vi "sub_result-update.vi"   [LabVIEW 2019]
uses:
  _ctrl/rw.ctl
  SubVIs/common/_ctrl/system-status.ctl
  SubVIs/common/Glob_Ref.vi
types:
  T1 = typedef "rw.ctl" = enum16{"read", "write"}
  T2 = typedef "DL950_wfms.ctl" = cluster{"wfms":waveform(dbl)[], "Waveform_2":cluster{"t0":dbl, "dt":dbl, "Y":dbl[][]}, "items":dbl[][], "da950_array":dbl[]}
  T3 = typedef "Testing-info.ctl" = cluster{"전체채널수":u8, "현재채널번호":u8, "Irms":dbl, "입력전압":dbl, "입력전류":dbl, "출력전압":dbl, "출력전류":dbl, "온도":dbl, "제어단 단선":bool, "제어단 단락":bool, "제어단 특성변화":bool, "출력단 단선":bool, "출력단 단락":bool, "출력단 특성변화":bool, "출력단 전압":bool, "카운트 일치":bool, "Irms 판정":bool, "온도":bool, "테스트 회수":u32, "TestType":T4, "현재회수":u32, "Ch selection":cluster{"1ch":bool, "2ch":bool, "3ch":bool, "4ch":bool, "5ch":bool, "6ch":bool}, "반복":u32, "Path":path, "파일생성주기":u32, "start time":dbl, "stop time":dbl, "현재반복회수":u32, "NG":cluster{"입출력 카운트":bool, "출력전류RMS":bool}}
  T4 = typedef "sequence_single.ctl" = enum16{"Register", "RC", "B1", "B2", "B3", "Oper_LV", "Oper_HV", "ContR_LV"}
  T5 = typedef "system-status.ctl" = enum16{"Initial", "Update", "Clear", "Read"}
  T6 = typedef "measure_reg.ctl" = cluster{"입력카운트":dbl, "출력카운트":dbl, "부하전압 RMS":dbl, "입력전류 RMS":dbl, "출력전류 RMS":dbl, "온도":dbl, "부하전압(고장)":dbl}
  T7 = typedef "measure_rc.ctl" = cluster{"입력카운트":dbl, "출력카운트":dbl, "Rising Time 63%":dbl, "Rising Time 98%":dbl, "Failing Time 37%":dbl, "입력전류 RMS":dbl, "출력전류 RMS":dbl, "출력전압 + 평균 63%":dbl, "출력전압 - 평균 63%":dbl, "출력전류 평균 63%":dbl, "접촉저항":dbl, "온도":dbl, "충전전압 63초":dbl, "충전전압 98초":dbl, "충전전류 37초":dbl, "방전전압":dbl, "전압강하":dbl, "부하전압(고장)":dbl}
  T8 = typedef "data_contR.ctl" = cluster{"입력카운트":dbl, "출력카운트":dbl, "입력전류 RMS":dbl, "출력전류 RMS":dbl, "출력전압(+)_Avg":dbl, "출력전압(-)_Avg":dbl, "출력전류_Avg":dbl, "접촉저항":dbl, "온도":dbl, "부하전압":dbl}
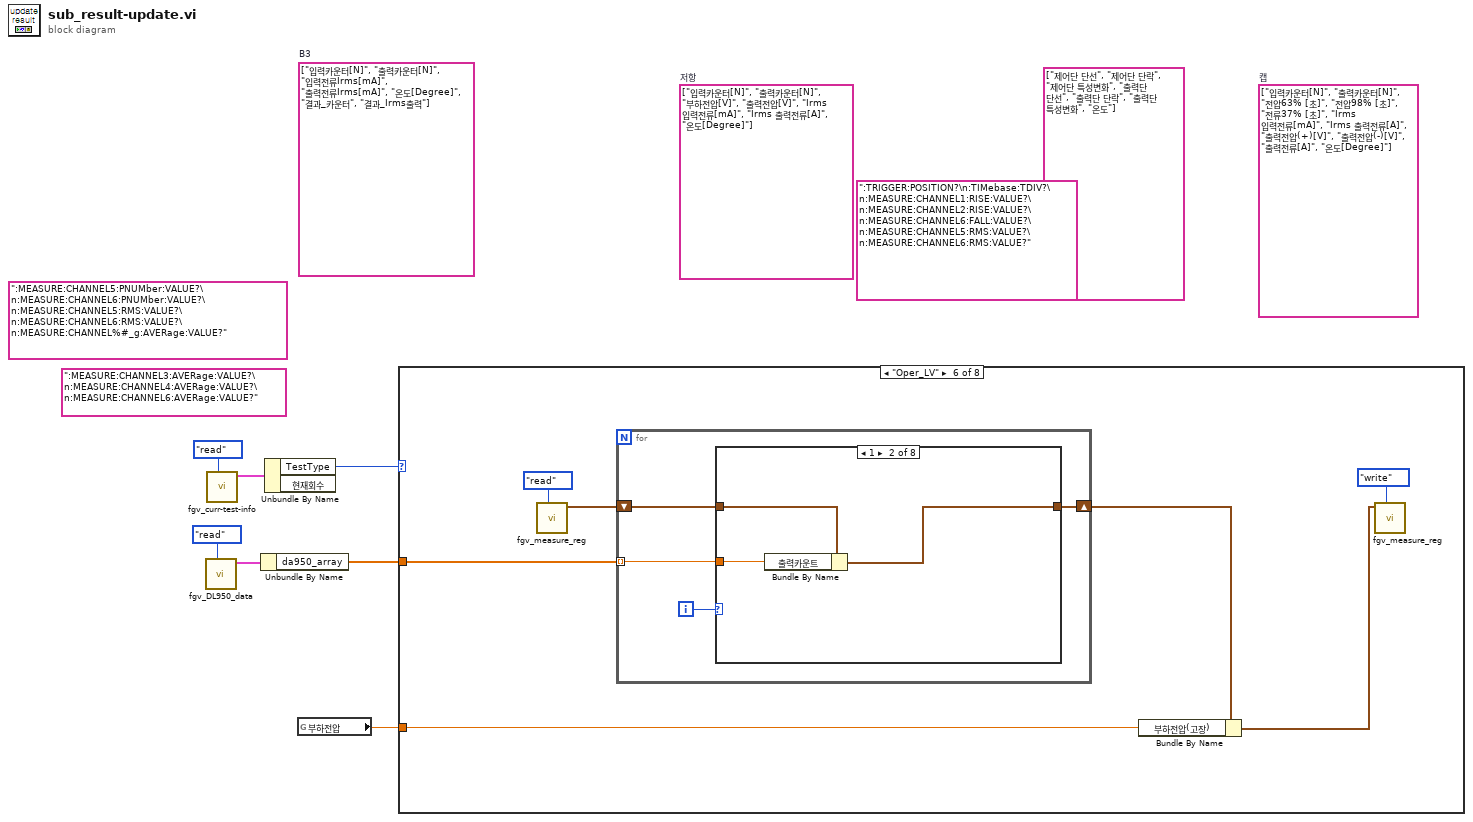
[diagram p0: block diagram]
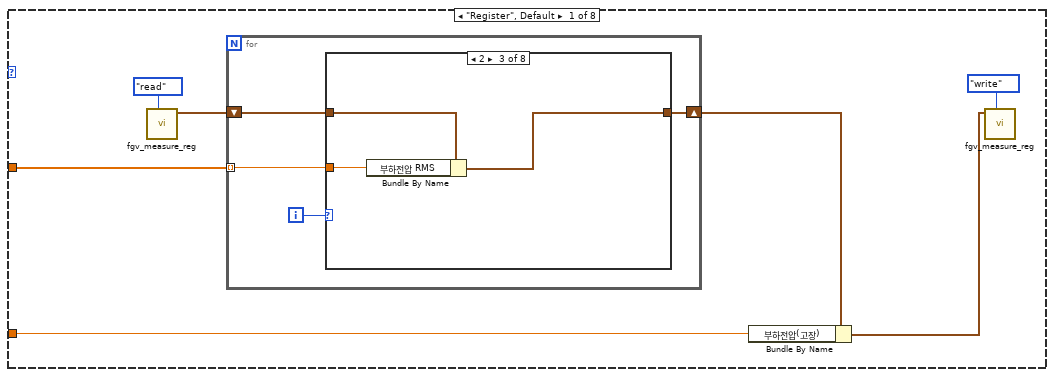
[diagram p2: hidden frame]
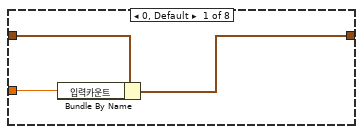
[diagram p3: hidden frame]
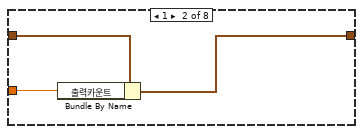
[diagram p4: hidden frame]
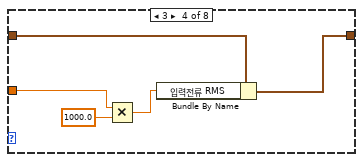
[diagram p5: hidden frame]
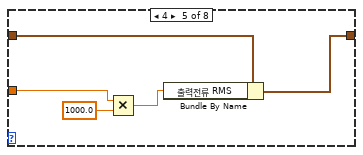
[diagram p6: hidden frame]
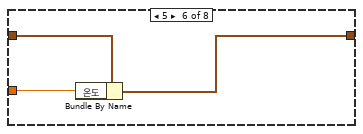
[diagram p7: hidden frame]
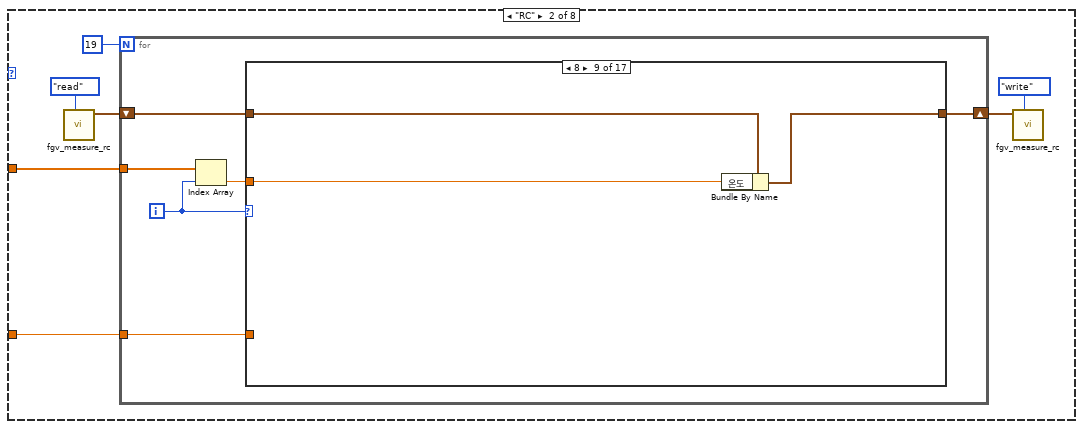
[diagram p10: hidden frame]
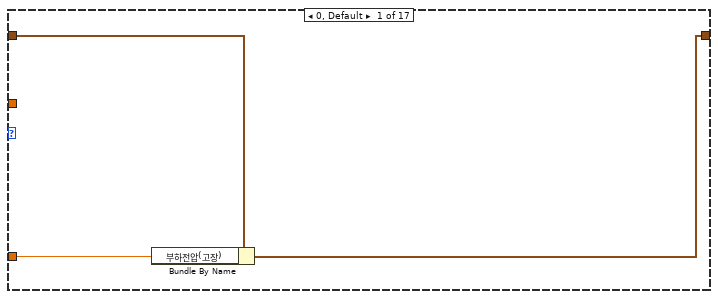
[diagram p11: hidden frame]
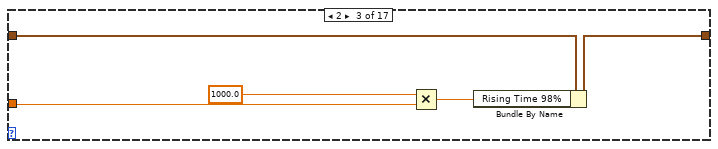
[diagram p13: hidden frame]
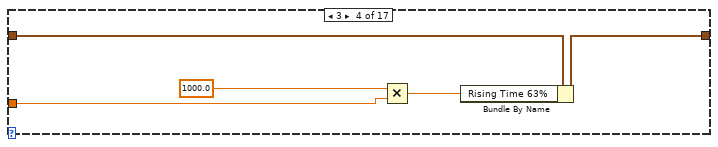
[diagram p14: hidden frame]
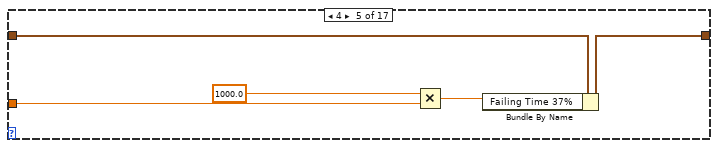
[diagram p15: hidden frame]
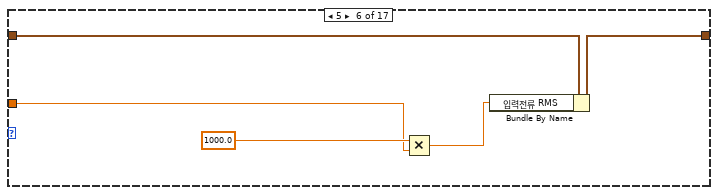
[diagram p16: hidden frame]
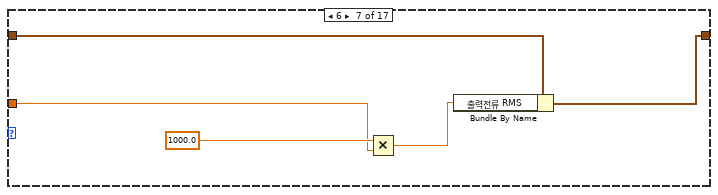
[diagram p17: hidden frame]
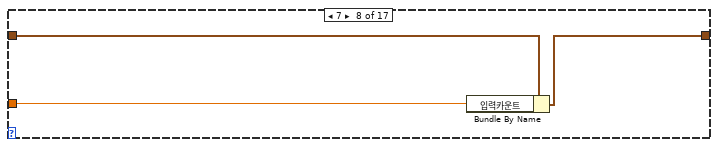
[diagram p18: hidden frame]
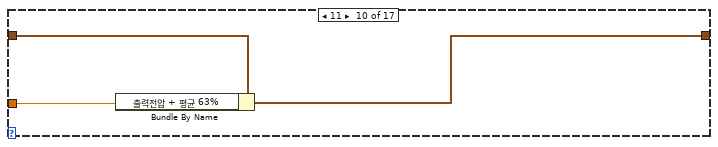
[diagram p19: hidden frame]
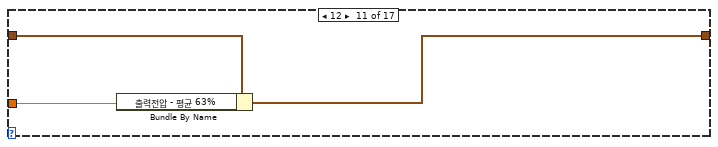
[diagram p20: hidden frame]
diagram:
  (unwired) ":MEASURE:CHANNEL3:AVERage:VALUE?\n:MEASURE:CHANNEL4:AVERage:VALUE?\n:MEASURE:CHANNEL6:AVERage:VALUE?" ("String")
  (unwired) ":MEASURE:CHANNEL5:PNUMber:VALUE?\n:MEASURE:CHANNEL6:PNUMber:VALUE?\n:MEASURE:CHANNEL5:RMS:VALUE?\n:MEASURE:CHANNEL6:RMS:VALUE?\n:MEASURE:CHANNEL%#_g:AVERage:VALUE?" ("String")
  (unwired) string[] ["입력카운터[N]", "출력카운터[N]", "입력전류Irms[mA]", "출력전류Irms[mA]", "온도[Degree]", "결과_카운터", "결과_Irms출력"]  # B3
  (unwired) ":TRIGGER:POSITION?\n:TIMebase:TDIV?\n:MEASURE:CHANNEL1:RISE:VALUE?\n:MEASURE:CHANNEL2:RISE:VALUE?\n:MEASURE:CHANNEL6:FALL:VALUE?\n:MEASURE:CHANNEL5:RMS:VALUE?\n:MEASURE:CHANNEL6:RMS:VALUE?" ("String")
  (unwired) string[] ["제어단 단선", "제어단 단락", "제어단 특성변화", "출력단 단선", "출력단 단락", "출력단 특성변화", "온도"] ("Column Header Strings[]")
  (unwired) string[] ["입력카운터[N]", "출력카운터[N]", "전압63% [초]", "전압98% [초]", "전류37% [초]", "Irms 입력전류[mA]", "Irms 출력전류[A]", "출력전압(+)[V]", "출력전압(-)[V]", "출력전류[A]", "온도[Degree]"]  # 캡
  (unwired) string[] ["입력카운터[N]", "출력카운터[N]", "부하전압[V]", "출력전압[V]", "Irms 입력전류[mA]", "Irms 출력전류[A]", "온도[Degree]"]  # 저항
  n1 = call "fgv_DL950_data.vi"("cmd"=rw."read") -> ("DL950 wfm 2"=w3:T2)  [unwired: 9 in, 1 out]
  n2 = call "fgv_curr-test-info.vi"("cmd"=rw."read") -> ("현재테스트 정보 2"=w5:T3)  [unwired: 10 in]
  n3 = Unbundle By Name(w3) -> ("da950_array"=w4:dbl[])
  n4 = Unbundle By Name(w5) -> ("TestType"=w7:T4)  [unwired: 1 out]
  n5 = global read "Glob_Ref.vi" "부하전압"() -> (w1:dbl)
  n6 = case shown="\"Oper_LV\"" w7 {
    tunnel: w4 -> [w14 w47 w132 w218 w253 w288 w331 w376]
    tunnel: w1 -> [w8 w43 w128 w212 w248 w282 w330 w372]
    frame "Register", Default {
      n7 = call "fgv_measure_reg.vi"("cmd"=rw."read") -> ("measure_reg 2"=w12:T6)  [unwired: 10 in]
      n8 = for {
        tunnel: w14 -> [w15] mode=indexing
        shift-right: [w16] -> w10
        shift-left: w12 -> [w17]
        i -> [w18]
        n9 = case shown="2" w18 {
          tunnel: w17 -> [w21 w24 w27 w32 w37 w40 w41 w42]
          tunnel: [w20 w23 w26 w31 w36 w39 w41 w42] -> w16
          tunnel: w15 -> [w19 w22 w25 w30 w34 w38 _ _]
          frame 0, Default {
            n10 = Bundle By Name(cluster=w21, "입력카운트"=w19) -> (w20:T6)
          }
          frame 1 {
            n11 = Bundle By Name(cluster=w24, "출력카운트"=w22) -> (w23:T6)
          }
          frame 2 {
            n12 = Bundle By Name(cluster=w27, "부하전압 RMS"=w25) -> (w26:T6)
          }
          frame 3 {
            n13 = Multiply(x=w30, y=1000.0) -> (x*y=w29:dbl)
            n14 = Bundle By Name(cluster=w32, "입력전류 RMS"=w29) -> (w31:T6)
          }
          frame 4 {
            n15 = Multiply(x=w34, y=1000.0) -> (x*y=w33:dbl)
            n16 = Bundle By Name(cluster=w37, "출력전류 RMS"=w33) -> (w36:T6)
          }
          frame 5 {
            n17 = Bundle By Name(cluster=w40, "온도"=w38) -> (w39:T6)
          }
          frame 6 {
          }
          frame 7 {
          }
        }
      }
      n18 = Bundle By Name(cluster=w10, "부하전압(고장)"=w8) -> (w9:T6)
      n19 = call "fgv_measure_reg.vi"("cmd"=rw."write", "measure_reg"=w9) -> ()  [unwired: 9 in, 1 out]
    }
    frame "RC" {
      n20 = call "fgv_measure_rc.vi"("cmd"=rw."read") -> ("measure_rc 2"=w46:T7)  [unwired: 10 in]
      n21 = for {
        N: 19 -> [_]
        tunnel: w47 -> [w55]
        shift-right: [w50] -> w45
        shift-left: w46 -> [w54]
        tunnel: w43 -> [w51]
        i -> [w52]
        n22 = Index Array(array=w55, index=w52) -> (element=w53:dbl)
        n23 = case shown="8" w52 {
          tunnel: w54 -> [w58 w59 w64 w69 w74 w79 w81 w87 w90 w92 w95 w98 w104 w105 w106 w124 w127]
          tunnel: [w57 w59 w63 w68 w73 w78 w80 w86 w89 w91 w94 w97 w103 w105 w106 w125 w127] -> w50
          tunnel: w53 -> [_ _ w62 w66 w71 w76 w82 w85 w88 w93 w96 w99 _ _ _ _ _]
          tunnel: w51 -> [w56 _ _ _ _ _ _ _ _ _ _ _ _ _ _ _ _]
          frame 0, Default {
            n24 = Bundle By Name(cluster=w58, "부하전압(고장)"=w56) -> (w57:T7)
          }
          frame 1 {
          }
          frame 2 {
            n25 = Multiply(x=1000.0, y=w62) -> (x*y=w61:dbl)
            n26 = Bundle By Name(cluster=w64, "Rising Time 98%"=w61) -> (w63:T7)
          }
          frame 3 {
            n27 = Multiply(x=1000.0, y=w66) -> (x*y=w65:dbl)
            n28 = Bundle By Name(cluster=w69, "Rising Time 63%"=w65) -> (w68:T7)
          }
          frame 4 {
            n29 = Multiply(x=1000.0, y=w71) -> (x*y=w70:dbl)
            n30 = Bundle By Name(cluster=w74, "Failing Time 37%"=w70) -> (w73:T7)
          }
          frame 5 {
            n31 = Multiply(x=1000.0, y=w76) -> (x*y=w75:dbl)
            n32 = Bundle By Name(cluster=w79, "입력전류 RMS"=w75) -> (w78:T7)
          }
          frame 6 {
            n33 = Multiply(x=1000.0, y=w82) -> (x*y=w83:dbl)
            n34 = Bundle By Name(cluster=w81, "출력전류 RMS"=w83) -> (w80:T7)
          }
          frame 7 {
            n35 = Bundle By Name(cluster=w87, "입력카운트"=w85) -> (w86:T7)
          }
          frame 8 {
            n36 = Bundle By Name(cluster=w90, "온도"=w88) -> (w89:T7)
          }
          frame 11 {
            n37 = Bundle By Name(cluster=w92, "출력전압 + 평균 63%"=w93) -> (w91:T7)
          }
          frame 12 {
            n38 = Bundle By Name(cluster=w95, "출력전압 - 평균 63%"=w96) -> (w94:T7)
          }
          frame 13 {
            n39 = Bundle By Name(cluster=w98, "출력전류 평균 63%"=w99) -> (w97:T7)
          }
          frame 14 {
            n40 = call "fgv_AI.vi"("Mode"=system-status."Read") -> ("mean-vals"=w101:dbl[])  [unwired: 8 in, 2 out]
            n41 = Index Array(array=w101) -> (element=w100:dbl)  [unwired: 1 in]
            n42 = Bundle By Name(cluster=w104, "방전전압"=w100) -> (w103:T7)
          }
          frame 15 {
          }
          frame 16 {
          }
          frame 18 {
            n43 = Unbundle By Name(w124) -> ("출력전압 + 평균 63%"=w112:dbl, "출력전압 - 평균 63%"=w109:dbl, "출력전류 평균 63%"=w116:dbl)
            n44 = Number To Fractional String(number=w109) -> (F-format string=w111:string)  [unwired: 3 in]
            n45 = Number To Fractional String(number=w112) -> (F-format string=w113:string)  [unwired: 3 in]
            n46 = call "sub_log_basic.vi"("desc"=w113, "Title"="output volt+ 63%") -> ("error out"=w108:errorcluster)  [unwired: 9 in]
            n47 = call "sub_log_basic.vi"("error in"=w108, "desc"=w111, "Title"="output volt- 63%") -> ("error out"=w107:errorcluster)  [unwired: 8 in]
            n48 = Subtract(x=w112, y=w109) -> (x-y=w126:dbl)
            n49 = Divide(x=w126, y=w116) -> (x/y=w122:dbl)
            n50 = Number To Fractional String(number=w116) -> (F-format string=w118:string)  [unwired: 3 in]
            n51 = Multiply(x=1000.0, y=w122) -> (x*y=w120:dbl)
            n52 = call "sub_log_basic.vi"("error in"=w107, "desc"=w118, "Title"="output current 63%") -> ("error out"=w115:errorcluster)  [unwired: 8 in]
            n53 = Bundle By Name(cluster=w124, "접촉저항"=w120) -> (w125:T7)
            n54 = Number To Fractional String(number=w120) -> (F-format string=w119:string)  [unwired: 3 in]
            n55 = call "sub_log_basic.vi"("error in"=w115, "desc"=w119, "Title"="contact register") -> ()  [unwired: 8 in, 1 out]
          }
          frame 19 {
          }
        }
      }
      n56 = call "fgv_measure_rc.vi"("cmd"=rw."write", "measure_rc"=w45) -> ()  [unwired: 9 in, 1 out]
    }
    frame "B1" {
      n57 = call "fgv_measure_rc.vi"("cmd"=rw."read") -> ("measure_rc 2"=w131:T7)  [unwired: 10 in]
      n58 = for {
        N: 19 -> [_]
        tunnel: w132 -> [w138]
        shift-right: [w139] -> w130
        shift-left: w131 -> [w140]
        tunnel: w128 -> [w135]
        i -> [w137]
        n59 = Index Array(array=w138, index=w137) -> (element=w136:dbl)
        n60 = case shown="0, Default" w137 {
          tunnel: w140 -> [w143 w144 w149 w154 w159 w164 w166 w172 w174 w177 w180 w186 w188 w190 w208 w211]
          tunnel: [w141 w144 w148 w153 w158 w163 w165 w171 w173 w176 w179 w185 w187 w190 w209 w211] -> w139
          tunnel: w136 -> [_ _ w147 w151 w156 w161 w167 w170 w175 w178 w181 _ w189 _ _ _]
          tunnel: w135 -> [w142 _ _ _ _ _ _ _ _ _ _ _ _ _ _ _]
          frame 0, Default {
            n61 = Bundle By Name(cluster=w143, "부하전압(고장)"=w142) -> (w141:T7)
          }
          frame 1 {
          }
          frame 2 {
            n62 = Multiply(x=1000.0, y=w147) -> (x*y=w146:dbl)
            n63 = Bundle By Name(cluster=w149, "Rising Time 98%"=w146) -> (w148:T7)
          }
          frame 3 {
            n64 = Multiply(x=1000.0, y=w151) -> (x*y=w150:dbl)
            n65 = Bundle By Name(cluster=w154, "Rising Time 63%"=w150) -> (w153:T7)
          }
          frame 4 {
            n66 = Multiply(x=1000.0, y=w156) -> (x*y=w155:dbl)
            n67 = Bundle By Name(cluster=w159, "Failing Time 37%"=w155) -> (w158:T7)
          }
          frame 5 {
            n68 = Multiply(x=1000.0, y=w161) -> (x*y=w160:dbl)
            n69 = Bundle By Name(cluster=w164, "입력전류 RMS"=w160) -> (w163:T7)
          }
          frame 6 {
            n70 = Multiply(x=1000.0, y=w167) -> (x*y=w168:dbl)
            n71 = Bundle By Name(cluster=w166, "출력전류 RMS"=w168) -> (w165:T7)
          }
          frame 7 {
            n72 = Bundle By Name(cluster=w172, "입력카운트"=w170) -> (w171:T7)
          }
          frame 10 {
            n73 = Bundle By Name(cluster=w174, "출력전압 + 평균 63%"=w175) -> (w173:T7)
          }
          frame 11 {
            n74 = Bundle By Name(cluster=w177, "출력전압 - 평균 63%"=w178) -> (w176:T7)
          }
          frame 12 {
            n75 = Bundle By Name(cluster=w180, "출력전류 평균 63%"=w181) -> (w179:T7)
          }
          frame 13 {
            n76 = call "fgv_AI.vi"("Mode"=system-status."Read") -> ("mean-vals"=w183:dbl[])  [unwired: 8 in, 2 out]
            n77 = Index Array(array=w183) -> (element=w182:dbl)  [unwired: 1 in]
            n78 = Bundle By Name(cluster=w186, "방전전압"=w182) -> (w185:T7)
          }
          frame 15 {
            n79 = Bundle By Name(cluster=w188, "온도"=w189) -> (w187:T7)
          }
          frame 16 {
          }
          frame 18 {
            n80 = Unbundle By Name(w208) -> ("출력전압 + 평균 63%"=w196:dbl, "출력전압 - 평균 63%"=w193:dbl, "출력전류 평균 63%"=w200:dbl)
            n81 = Number To Fractional String(number=w193) -> (F-format string=w195:string)  [unwired: 3 in]
            n82 = Number To Fractional String(number=w196) -> (F-format string=w197:string)  [unwired: 3 in]
            n83 = call "sub_log_basic.vi"("desc"=w197, "Title"="output volt+ 63%") -> ("error out"=w192:errorcluster)  [unwired: 9 in]
            n84 = call "sub_log_basic.vi"("error in"=w192, "desc"=w195, "Title"="output volt- 63%") -> ("error out"=w191:errorcluster)  [unwired: 8 in]
            n85 = Subtract(x=w196, y=w193) -> (x-y=w210:dbl)
            n86 = Divide(x=w210, y=w200) -> (x/y=w206:dbl)
            n87 = Number To Fractional String(number=w200) -> (F-format string=w202:string)  [unwired: 3 in]
            n88 = Multiply(x=1000.0, y=w206) -> (x*y=w204:dbl)
            n89 = call "sub_log_basic.vi"("error in"=w191, "desc"=w202, "Title"="output current 63%") -> ("error out"=w199:errorcluster)  [unwired: 8 in]
            n90 = Bundle By Name(cluster=w208, "접촉저항"=w204) -> (w209:T7)
            n91 = Number To Fractional String(number=w204) -> (F-format string=w203:string)  [unwired: 3 in]
            n92 = call "sub_log_basic.vi"("error in"=w199, "desc"=w203, "Title"="contact register") -> ()  [unwired: 8 in, 1 out]
          }
          frame 19 {
          }
        }
      }
      n93 = call "fgv_measure_rc.vi"("cmd"=rw."write", "measure_rc"=w130) -> ()  [unwired: 9 in, 1 out]
    }
    frame "B2" {
      n94 = call "fgv_measure_reg.vi"("cmd"=rw."read") -> ("measure_reg 2"=w216:T6)  [unwired: 10 in]
      n95 = for {
        tunnel: w218 -> [w219] mode=indexing
        shift-right: [w220] -> w214
        shift-left: w216 -> [w221]
        i -> [w222]
        n96 = case shown="2" w222 {
          tunnel: w221 -> [w225 w228 w231 w236 w241 w244 w245 w246]
          tunnel: [w224 w227 w230 w235 w240 w243 w245 w246] -> w220
          tunnel: w219 -> [w223 w226 w229 w234 w238 w242 _ _]
          frame 0, Default {
            n97 = Bundle By Name(cluster=w225, "입력카운트"=w223) -> (w224:T6)
          }
          frame 1 {
            n98 = Bundle By Name(cluster=w228, "출력카운트"=w226) -> (w227:T6)
          }
          frame 2 {
            n99 = Bundle By Name(cluster=w231, "부하전압 RMS"=w229) -> (w230:T6)
          }
          frame 3 {
            n100 = Multiply(x=w234, y=1000.0) -> (x*y=w233:dbl)
            n101 = Bundle By Name(cluster=w236, "입력전류 RMS"=w233) -> (w235:T6)
          }
          frame 4 {
            n102 = Multiply(x=w238, y=1000.0) -> (x*y=w237:dbl)
            n103 = Bundle By Name(cluster=w241, "출력전류 RMS"=w237) -> (w240:T6)
          }
          frame 5 {
            n104 = Bundle By Name(cluster=w244, "온도"=w242) -> (w243:T6)
          }
          frame 6 {
          }
          frame 7 {
          }
        }
      }
      n105 = Bundle By Name(cluster=w214, "부하전압(고장)"=w212) -> (w213:T6)
      n106 = call "fgv_measure_reg.vi"("cmd"=rw."write", "measure_reg"=w213) -> ()  [unwired: 9 in, 1 out]
    }
    frame "B3" {
      n107 = call "fgv_measure_reg.vi"("cmd"=rw."read") -> ("measure_reg 2"=w251:T6)  [unwired: 10 in]
      n108 = for {
        tunnel: w253 -> [w254] mode=indexing
        shift-right: [w255] -> w249
        shift-left: w251 -> [w256]
        i -> [w257]
        n109 = case shown="0, Default" w257 {
          tunnel: w256 -> [w260 w263 w266 w271 w276 w279 w280 w281]
          tunnel: [w259 w262 w265 w270 w275 w278 w280 w281] -> w255
          tunnel: w254 -> [w258 w261 w264 w269 w273 w277 _ _]
          frame 0, Default {
            n110 = Bundle By Name(cluster=w260, "입력카운트"=w258) -> (w259:T6)
          }
          frame 1 {
            n111 = Bundle By Name(cluster=w263, "출력카운트"=w261) -> (w262:T6)
          }
          frame 2 {
            n112 = Bundle By Name(cluster=w266, "부하전압 RMS"=w264) -> (w265:T6)
          }
          frame 3 {
            n113 = Multiply(x=w269, y=1000.0) -> (x*y=w268:dbl)
            n114 = Bundle By Name(cluster=w271, "입력전류 RMS"=w268) -> (w270:T6)
          }
          frame 4 {
            n115 = Multiply(x=w273, y=1000.0) -> (x*y=w272:dbl)
            n116 = Bundle By Name(cluster=w276, "출력전류 RMS"=w272) -> (w275:T6)
          }
          frame 5 {
            n117 = Bundle By Name(cluster=w279, "온도"=w277) -> (w278:T6)
          }
          frame 6 {
          }
          frame 7 {
          }
        }
      }
      n118 = Bundle By Name(cluster=w249, "부하전압(고장)"=w248) -> (w247:T6)
      n119 = call "fgv_measure_reg.vi"("cmd"=rw."write", "measure_reg"=w247) -> ()  [unwired: 9 in, 1 out]
    }
    frame "Oper_LV" {
      n120 = call "fgv_measure_reg.vi"("cmd"=rw."read") -> ("measure_reg 2"=w286:T6)  [unwired: 10 in]
      n121 = for {
        tunnel: w288 -> [w289] mode=indexing
        shift-right: [w290] -> w284
        shift-left: w286 -> [w291]
        i -> [w292]
        n122 = case shown="1" w292 {
          tunnel: w291 -> [w295 w298 w301 w306 w311 w314 w315 w316]
          tunnel: [w294 w297 w300 w305 w310 w313 w315 w316] -> w290
          tunnel: w289 -> [w293 w296 w299 w304 w308 w312 _ _]
          frame 0, Default {
            n123 = Bundle By Name(cluster=w295, "입력카운트"=w293) -> (w294:T6)
          }
          frame 1 {
            n124 = Bundle By Name(cluster=w298, "출력카운트"=w296) -> (w297:T6)
          }
          frame 2 {
            n125 = Bundle By Name(cluster=w301, "부하전압 RMS"=w299) -> (w300:T6)
          }
          frame 3 {
            n126 = Multiply(x=w304, y=1000.0) -> (x*y=w303:dbl)
            n127 = Bundle By Name(cluster=w306, "입력전류 RMS"=w303) -> (w305:T6)
          }
          frame 4 {
            n128 = Multiply(x=w308, y=1000.0) -> (x*y=w307:dbl)
            n129 = Bundle By Name(cluster=w311, "출력전류 RMS"=w307) -> (w310:T6)
          }
          frame 5 {
            n130 = Bundle By Name(cluster=w314, "온도"=w312) -> (w313:T6)
          }
          frame 6 {
          }
          frame 7 {
          }
        }
      }
      n131 = Bundle By Name(cluster=w284, "부하전압(고장)"=w282) -> (w283:T6)
      n132 = call "fgv_measure_reg.vi"("cmd"=rw."write", "measure_reg"=w283) -> ()  [unwired: 9 in, 1 out]
    }
    frame "ContR_LV" {
      w318 = 1000.0 ("y")
      n133 = call "fgv_measure_ContR.vi"("cmd"=rw."read") -> ("measure_ContR Out"=w328:T8)  [unwired: 9 in, 1 out]
      n134 = for {
        tunnel: w331 -> [w332] mode=indexing
        shift-right: [w333] -> w325
        shift-left: w328 -> [w334]
        i -> [w335]
        n135 = case shown="11" w335 {
          tunnel: w334 -> [w338 w341 w346 w351 w354 w355 w356 w361 w366 w369 w370 w371]
          tunnel: [w337 w340 w345 w350 w353 w355 w356 w360 w365 w368 w370 w371] -> w333
          tunnel: w332 -> [w336 w339 w343 w349 w352 _ _ w358 w363 w367 _ _]
          frame 0, Default {
            n136 = Bundle By Name(cluster=w338, "입력카운트"=w336) -> (w337:T8)
          }
          frame 1 {
            n137 = Bundle By Name(cluster=w341, "출력카운트"=w339) -> (w340:T8)
          }
          frame 2 {
            n138 = Multiply(x=w343, y=1000.0) -> (x*y=w342:dbl)
            n139 = Bundle By Name(cluster=w346, "입력전류 RMS"=w342) -> (w345:T8)
          }
          frame 3 {
            n140 = Multiply(x=w349, y=1000.0) -> (x*y=w348:dbl)
            n141 = Bundle By Name(cluster=w351, "출력전류 RMS"=w348) -> (w350:T8)
          }
          frame 4 {
            n142 = Bundle By Name(cluster=w354, "온도"=w352) -> (w353:T8)
          }
          frame 5 {
          }
          frame 6 {
          }
          frame 7 {
            n143 = Multiply(x=w358, y=1000.0) -> (x*y=w357:dbl)
            n144 = Bundle By Name(cluster=w361, "출력전압(+)_Avg"=w357) -> (w360:T8)
          }
          frame 8 {
            n145 = Multiply(x=w363, y=1000.0) -> (x*y=w362:dbl)
            n146 = Bundle By Name(cluster=w366, "출력전압(-)_Avg"=w362) -> (w365:T8)
          }
          frame 9 {
            n147 = Bundle By Name(cluster=w369, "출력전류_Avg"=w367) -> (w368:T8)
          }
          frame 10 {
          }
          frame 11 {
          }
        }
      }
      n148 = Unbundle By Name(w325) -> ("출력전압(+)_Avg"=w324:dbl, "출력전압(-)_Avg"=w323:dbl, "출력전류_Avg"=w321:dbl)
      n149 = Multiply(x=w321, y=w318) -> (x*y=w320:dbl)
      n150 = Subtract(x=w324, y=w323) -> (x-y=w322:dbl)
      n151 = Divide(x=w322, y=w320) -> (x/y=w319:dbl)
      n152 = Multiply(x=w319, y=w318) -> (x*y=w317:dbl)
      n153 = Bundle By Name(cluster=w325, "접촉저항"=w317, "출력전압(-)_Avg"=w330) -> (w326:T8)
      n154 = call "fgv_measure_ContR.vi"("cmd"=rw."write", "measure_ContR In"=w326) -> ()  [unwired: 8 in, 2 out]
    }
    frame "Oper_HV" {
      n155 = call "fgv_measure_rc.vi"("cmd"=rw."read") -> ("measure_rc 2"=w375:T7)  [unwired: 10 in]
      n156 = for {
        N: 19 -> [_]
        tunnel: w376 -> [w384]
        shift-right: [w379] -> w374
        shift-left: w375 -> [w383]
        tunnel: w372 -> [w380]
        i -> [w381]
        n157 = Index Array(array=w384, index=w381) -> (element=w382:dbl)
        n158 = case shown="8" w381 {
          tunnel: w383 -> [w387 w388 w393 w398 w403 w408 w410 w416 w419 w421 w424 w427 w433 w434 w435 w453 w456]
          tunnel: [w386 w388 w392 w397 w402 w407 w409 w415 w418 w420 w423 w426 w432 w434 w435 w454 w456] -> w379
          tunnel: w382 -> [_ _ w391 w395 w400 w405 w411 w414 w417 w422 w425 w428 _ _ _ _ _]
          tunnel: w380 -> [w385 _ _ _ _ _ _ _ _ _ _ _ _ _ _ _ _]
          frame 0, Default {
            n159 = Bundle By Name(cluster=w387, "부하전압(고장)"=w385) -> (w386:T7)
          }
          frame 1 {
          }
          frame 2 {
            n160 = Multiply(x=1000.0, y=w391) -> (x*y=w390:dbl)
            n161 = Bundle By Name(cluster=w393, "Rising Time 98%"=w390) -> (w392:T7)
          }
          frame 3 {
            n162 = Multiply(x=1000.0, y=w395) -> (x*y=w394:dbl)
            n163 = Bundle By Name(cluster=w398, "Rising Time 63%"=w394) -> (w397:T7)
          }
          frame 4 {
            n164 = Multiply(x=1000.0, y=w400) -> (x*y=w399:dbl)
            n165 = Bundle By Name(cluster=w403, "Failing Time 37%"=w399) -> (w402:T7)
          }
          frame 5 {
            n166 = Multiply(x=1000.0, y=w405) -> (x*y=w404:dbl)
            n167 = Bundle By Name(cluster=w408, "입력전류 RMS"=w404) -> (w407:T7)
          }
          frame 6 {
            n168 = Multiply(x=1000.0, y=w411) -> (x*y=w412:dbl)
            n169 = Bundle By Name(cluster=w410, "출력전류 RMS"=w412) -> (w409:T7)
          }
          frame 7 {
            n170 = Bundle By Name(cluster=w416, "입력카운트"=w414) -> (w415:T7)
          }
          frame 8 {
            n171 = Bundle By Name(cluster=w419, "온도"=w417) -> (w418:T7)
          }
          frame 11 {
            n172 = Bundle By Name(cluster=w421, "출력전압 + 평균 63%"=w422) -> (w420:T7)
          }
          frame 12 {
            n173 = Bundle By Name(cluster=w424, "출력전압 - 평균 63%"=w425) -> (w423:T7)
          }
          frame 13 {
            n174 = Bundle By Name(cluster=w427, "출력전류 평균 63%"=w428) -> (w426:T7)
          }
          frame 14 {
            n175 = call "fgv_AI.vi"("Mode"=system-status."Read") -> ("mean-vals"=w430:dbl[])  [unwired: 8 in, 2 out]
            n176 = Index Array(array=w430) -> (element=w429:dbl)  [unwired: 1 in]
            n177 = Bundle By Name(cluster=w433, "방전전압"=w429) -> (w432:T7)
          }
          frame 15 {
          }
          frame 16 {
          }
          frame 18 {
            n178 = Unbundle By Name(w453) -> ("출력전압 + 평균 63%"=w441:dbl, "출력전압 - 평균 63%"=w438:dbl, "출력전류 평균 63%"=w445:dbl)
            n179 = Number To Fractional String(number=w438) -> (F-format string=w440:string)  [unwired: 3 in]
            n180 = Number To Fractional String(number=w441) -> (F-format string=w442:string)  [unwired: 3 in]
            n181 = call "sub_log_basic.vi"("desc"=w442, "Title"="output volt+ 63%") -> ("error out"=w437:errorcluster)  [unwired: 9 in]
            n182 = call "sub_log_basic.vi"("error in"=w437, "desc"=w440, "Title"="output volt- 63%") -> ("error out"=w436:errorcluster)  [unwired: 8 in]
            n183 = Subtract(x=w441, y=w438) -> (x-y=w455:dbl)
            n184 = Divide(x=w455, y=w445) -> (x/y=w451:dbl)
            n185 = Number To Fractional String(number=w445) -> (F-format string=w447:string)  [unwired: 3 in]
            n186 = Multiply(x=1000.0, y=w451) -> (x*y=w449:dbl)
            n187 = call "sub_log_basic.vi"("error in"=w436, "desc"=w447, "Title"="output current 63%") -> ("error out"=w444:errorcluster)  [unwired: 8 in]
            n188 = Bundle By Name(cluster=w453, "접촉저항"=w449) -> (w454:T7)
            n189 = Number To Fractional String(number=w449) -> (F-format string=w448:string)  [unwired: 3 in]
            n190 = call "sub_log_basic.vi"("error in"=w444, "desc"=w448, "Title"="contact register") -> ()  [unwired: 8 in, 1 out]
          }
          frame 19 {
          }
        }
      }
      n191 = call "fgv_measure_rc.vi"("cmd"=rw."write", "measure_rc"=w374) -> ()  [unwired: 9 in, 1 out]
    }
  }
